vi "Test - Sensitivity.vi"(8 "error in (no error)":errorcluster, 9 "Step Frequency":dbl, 10 "Stop Frequency":dbl, 11 "Start Frequency":dbl) -> (0 "error out":errorcluster)   [LabVIEW 2020]
uses:
  Library - Test Executive.llb/Test Executive - Globals.vi
  Library - Test Executive.llb/Test Executive.lvlib
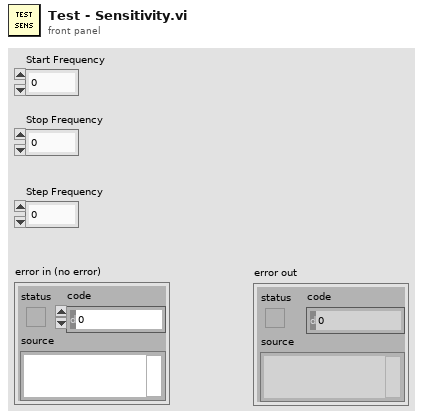
[diagram p1: front panel]
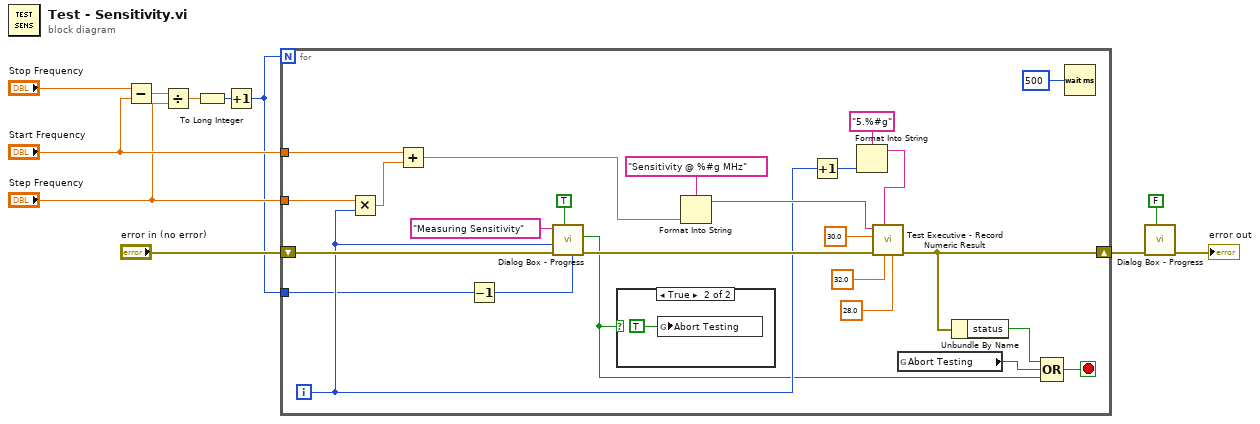
[diagram p0: block diagram]
diagram:
  n1 = Subtract(x="Stop Frequency", y="Start Frequency") -> (x-y=w9:dbl)
  n2 = Divide(x=w9, y="Step Frequency") -> (x/y=w8:dbl)
  n3 = To Long Integer(number=w8) -> (32bit integer=w5:i32)
  n4 = Increment(x=w5) -> (x+1=w1:i32)
  n5 = for {
    N: w1 -> [_]
    shift-right: [w17] -> w3
    shift-left: "error in (no error)" -> [w27]
    tunnel: "Start Frequency" -> [w25]
    tunnel: "Step Frequency" -> [w23]
    tunnel: w1 -> [w20]
    i -> [w21]
    stop <- w18 stop-if-true
    n6 = Multiply(x=w23, y=w21) -> (x*y=w24:dbl)
    n7 = Add(x=w25, y=w24) -> (x+y=w22:dbl)
    n8 = Decrement(x=w20) -> (x-1=w13:i32)
    n9 = call "Dialog Box - Progress.vi"("Text"="Measuring Sensitivity", "Bar Value"=w21, "error in (no error)"=w27, "Show"=TRUE, "Max Value (100)"=w13) -> ("Cancel"=w12:bool, "error out"=w26:errorcluster)  [unwired: 4 in]
    n10 = case shown="True" w12 {
      frame False {
      }
      frame True {
        n11 = global write "Test Executive - Globals.vi" "Abort Testing"(TRUE ("Abort Testing")) -> ()
      }
    }
    n12 = Format Into String(format string="Sensitivity @ %#g MHz", w22) -> (resulting string=w32:string)  [unwired: 2 in, 1 out]
    n13 = Increment(x=w21) -> (x+1=w30:i32)
    n14 = Format Into String(format string="5.%#g" ("Test Ref"), w30) -> (resulting string=w29:string)  [unwired: 2 in, 1 out]
    n15 = call "Test Executive - Record Numeric Result.vi"("Lower Limit"=28.0 ("Low Limit"), "Upper Limit"=32.0 ("High Limit"), "Test Ref"=w29, "error in (no error)"=w26, "Measurement"=30.0, "Test Name"=w32) -> ("error out"=w17:errorcluster)  [unwired: 5 in]
    n16 = global read "Test Executive - Globals.vi" "Abort Testing"() -> (w14:bool)
    n17 = Unbundle By Name(w17) -> ("status"=w16:bool)
    n18 = Compound Arithmetic op=OR(w16, w14, w12) -> (w18:bool)
    n19 = Wait (ms)(milliseconds to wait=u32 500) -> ()  [unwired: 1 out]
  }
  n20 = call "Dialog Box - Progress.vi"("error in (no error)"=w3, "Show"=FALSE) -> ("error out"=→"error out":errorcluster)  [unwired: 7 in, 1 out]
